vi "Sub_map.vi"(7 "error out":errorcluster, 10 "device":T2) -> (0 "error out 2":errorcluster caption="error out", 1 "x = y?":bool, 3 "device 2":T2)   [LabVIEW 2014]
panel:
  out "HID_SMBUS_S0":T1
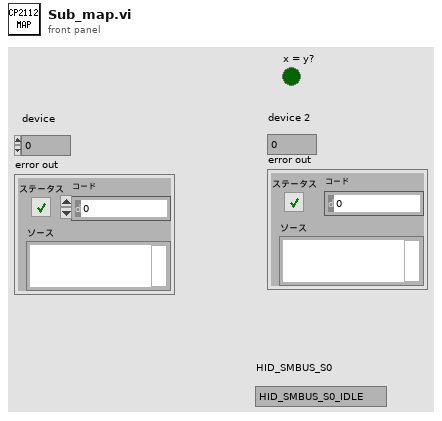
[diagram p1: front panel]
types:
  T1 = typedef "CP2112_SMBUS_S0.ctl" = enum8{"HID_SMBUS_S0_IDLE", "HID_SMBUS_S0_BUSY", "HID_SMBUS_S0_COMPLETE", "HID_SMBUS_S0_ERROR"}
  T2 = typedef "CP2112_device.ctl" = i32
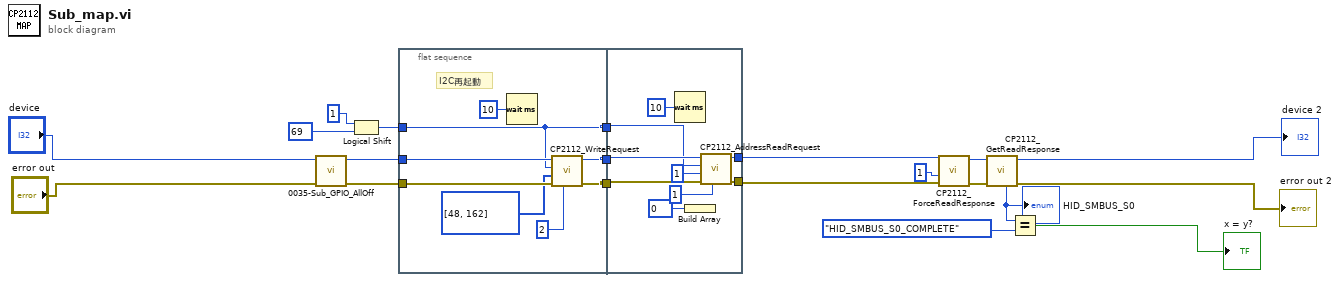
[diagram p0: block diagram]
diagram:
  n1 = call "0035-Sub_GPIO_AllOff.vi"("エラー出力 2"="error out", "device"="device") -> ("エラー出力"=w12:errorcluster, "deviceOut"=w13:T2)  [unwired: 8 in]
  n2 = Logical Shift(y=1, x=69) -> (x << y=w11:i32)
  n3 = flat-sequence {
    tunnel: w13 -> [w28]
    tunnel: w12 -> [w26]
    tunnel: w11 -> [w24]
    tunnel: [w27] -> w7
    tunnel: [w25] -> w6
    tunnel: [w24] -> w5
    tunnel: w7 -> [w33]
    tunnel: w6 -> [w34]
    tunnel: w5 -> [w32]
    tunnel: [w30] -> w4
    tunnel: [w29] -> w3
    frame #0 {
      # "I2C再起動"
      n4 = Wait (ms)(milliseconds to wait=u32 10 ("ミリ秒待機時間")) -> ()  [unwired: 1 out]
      n5 = call "CP2112_WriteRequest.vi"("numBytesToWrite"=u8 2, "error in (no error)"=w26, "buffer"=u8[] [48, 162], "slaveAddress"=w24, "device"=w28) -> ("error out"=w25:errorcluster, "deviceOut"=w27:T2)  [unwired: 4 in, 1 out]
    }
    frame #1 {
      n6 = Wait (ms)(milliseconds to wait=u32 10 ("ミリ秒待機時間")) -> ()  [unwired: 1 out]
      n7 = Build Array(u8 0 ("targetAddressSize")) -> ()  [unwired: 1 out]
      n8 = call "CP2112_AddressReadRequest.vi"("targetAddressSize"=u8 1, "error in (no error)"=w34, "numByteToRead"=i16 1, "slaveAddress"=w32, "device"=w33) -> ("error out"=w30:errorcluster, "deviceOut"=w29:T2)  [unwired: 4 in, 1 out]
    }
  }
  n9 = call "CP2112_ForceReadResponse.vi"("error in (no error)"=w4, "numByteToRead"=i16 1, "device"=w3) -> ("error out"=w18:errorcluster, "deviceOut"=w17:T2)  [unwired: 6 in, 1 out]
  n10 = call "CP2112_GetReadResponse.vi"("error in (no error)"=w18, "device"=w17) -> ("error out"=→"error out 2":errorcluster, "deviceOut"=→"device 2":T2, "HID_SMBUS_S0"=w14:T1)  [unwired: 4 in, 3 out]
  "HID_SMBUS_S0" <- w14
  n11 = Equal?(x=w14, y=CP2112_SMBUS_S0."HID_SMBUS_S0_COMPLETE" ("HID_SMBUS_S0")) -> (x = y?=→"x = y?":bool)
